vi "Firmware Wizard Check INI.vi"(8 "Error In":errorcluster) -> (0 "Error Out":errorcluster)   [LabVIEW 2011, in "LVH-LINX.lvlib"]
uses:
  LVH-LINX.lvlib
  <vilib>/LabVIEW Hacker/LVH-Toolbox/Common/LVH-Common.lvlib
  <vilib>/Utility/config.llb/NI_LVConfig.lvlib
  <vilib>/Utility/config.llb/Write Key (Path).vi
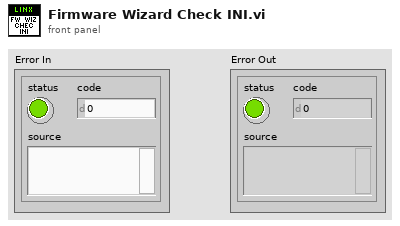
[diagram p1: front panel]
types:
  T1 = typedef "NI_LVConfig.lvlib/Config Data RefNum.ctl" = refnum<k1>
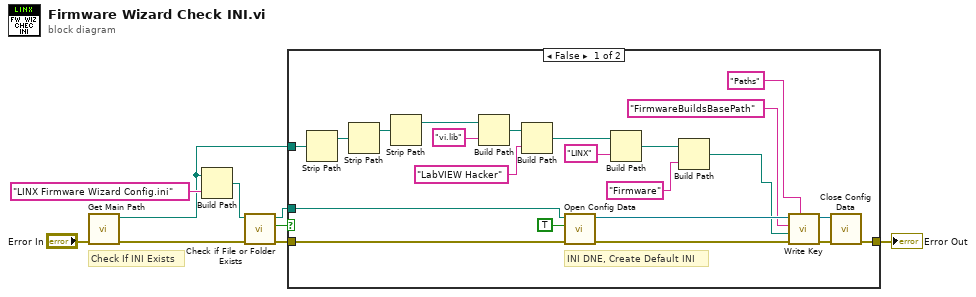
[diagram p0: block diagram]
diagram:
  # "Check If INI Exists"
  n1 = call <vilib>:"Get Main Path.vi"("Error In"="Error In") -> ("Error Out"=w9:errorcluster, "Main Dir"=w2:path)  [unwired: 8 in, 1 out]
  n2 = Build Path(base path=w2, name or relative path="LINX Firmware Wizard Config.ini") -> (appended path=w6:path)
  n3 = call <vilib>:"Check if File or Folder Exists.vi"("error in (no error)"=w9, "path"=w6) -> ("error out"=w5:errorcluster, "file or folder exists?"=w4:bool, "dup path"=w1:path)  [unwired: 7 in]
  n4 = case shown="False" w4 {
    tunnel: w5 -> [w24 w32]
    tunnel: [w21 w32] -> w3
    tunnel: w2 -> [w23 _]
    tunnel: w1 -> [w20 _]
    frame False {
      # "INI DNE, Create Default INI"
      n5 = Strip Path(path=w23) -> (stripped path=w19:path)  [unwired: 1 out]
      n6 = Strip Path(path=w19) -> (stripped path=w18:path)  [unwired: 1 out]
      n7 = Strip Path(path=w18) -> (stripped path=w17:path)  [unwired: 1 out]
      n8 = Build Path(base path=w17, name or relative path="vi.lib") -> (appended path=w15:path)
      n9 = Build Path(base path=w15, name or relative path="LabVIEW Hacker") -> (appended path=w13:path)
      n10 = call <vilib>:"Open Config Data.vi"("error in (no error)"=w24, "create file if necessary (T)"=TRUE, "configuration file path"=w20) -> ("error out"=w29:errorcluster, "refnum"=w28:T1)  [unwired: 6 in, 1 out]
      n11 = Build Path(base path=w13, name or relative path="LINX") -> (appended path=w11:path)
      n12 = Build Path(base path=w11, name or relative path="Firmware") -> (appended path=w10:path)
      n13 = call-poly <vilib>:"Write Key.vi"("section"="Paths", "error in (no error)"=w29, "value"=w10, "key"="FirmwareBuildsBasePath", "refnum"=w28) -> ("error out"=w30:errorcluster, "refnum out"=w31:T1)  [unwired: 4 in, 1 out]
      n14 = call <vilib>:"Close Config Data.vi"("error in (no error)"=w30, "refnum"=w31) -> ("error out"=w21:errorcluster)  [unwired: 8 in, 1 out]
    }
    frame True {
      # "INI Exists, Nothing To Do"
    }
  }
  "Error Out" <- w3
